vi "Parse Response JSON.vi"(8 "error in (no error)":errorcluster, 10 "Response JSON":string, 11 "RGetCurrentProgramScene in":refnum<class "RGetCurrentProgramScene.lvclass">) -> (0 "error out":errorcluster, 3 "RGetCurrentProgramScene out":refnum<class "RGetCurrentProgramScene.lvclass">)   [LabVIEW 2022 SP3, in "obs-websocket-lv.lvlib" / "RGetCurrentProgramScene.lvclass"]
uses:
  RGetCurrentProgramScene.lvclass
  RGetCurrentProgramScene.lvclass/RGetCurrentProgramScene.ctl
  <vilib>/IlluminatedG/lv-web-crypto/lv-json/JSON/JSON.lvlib
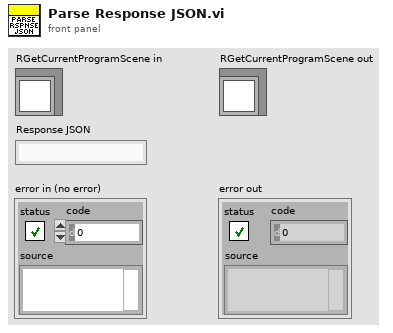
[diagram p1: front panel]
types:
  T1 = typedef "JSON.lvlib/JSON Item Type.ctl" = enum16{"unknown", "null", "Array", "Object", "String", "Number", "Boolean"}
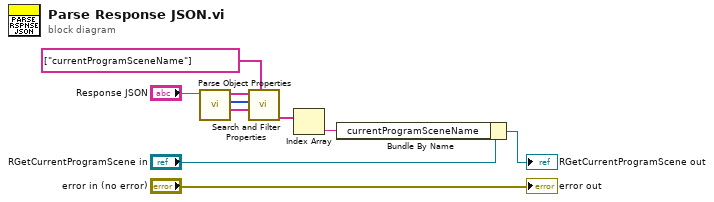
[diagram p0: block diagram]
diagram:
  n1 = call <vilib>:"Parse Object Properties.vi"("JSON String"="Response JSON") -> ("Values"=w5:string[], "Item Types"=w6:T1[], "Keys"=w7:string[])  [unwired: 7 in, 1 out]
  n2 = call <vilib>:"Search and Filter Properties.vi"("Search Keys"=string[] ["currentProgramSceneName"], "Values In"=w5, "Types In"=w6, "Keys In"=w7) -> ("Filtered Values"=w3:string[])  [unwired: 2 in, 5 out]
  n3 = Index Array(array=w3) -> (element=w1:string)  [unwired: 1 in]
  n4 = Bundle By Name(cluster="RGetCurrentProgramScene in", "currentProgramSceneName"=w1) -> (→"RGetCurrentProgramScene out":refnum<class "RGetCurrentProgramScene.lvclass">)
  "error out" <- "error in (no error)"
